vi "RunTest.vi"(8 "error in":errorcluster, 11 "Prueba31 in":refnum<class "Prueba31.lvclass">) -> (0 "error out":errorcluster, 2 "Resultado":string, 3 "Prueba31 out":refnum<class "Prueba31.lvclass">)   [LabVIEW 2019, in "Prueba31.lvclass"]
uses:
  Prueba31.lvclass
  Prueba31.lvclass/Prueba31.ctl
  QMH/Message Queue/Enqueue Message (Single).vi
  <vilib>/Utility/error.llb/Error Cluster From Error Code.vi
  RerenceAllControlsToolkit/_get control reference by name.vi
  <vilib>/ErrorRing/Error Ring.xnode
  QMH/Message Queue/Message Queue.lvlib
  QMH/User Event - Stop/User Event - Stop.lvlib
panel:
  in  "cb_frec_ext 2":string(combo)="31,5"
  in  "Tab Control":enum32{"externo", "interno"}(tab)
  out "cb_nivel_ext":dbl
  out "cb_frec_ext":dbl
  out "Tol - [dB]_ext":dbl
  out "Tol + [dB]_ext":dbl
  in  "generar_ext":bool
  out "cumple_ext":bool
  out "no_cumple_ext":bool
  out "frec_ref_ext":dbl
  out "nivel_ref_ext":dbl
  in  "señal_antes_ajuste_ext":dbl
  out "error_ext":dbl
  out "inc_expandida_ext":dbl
  in  "seguir_ext":bool
  out "voltaje_ext":dbl
  out "frecuencia_ext":dbl
  out "tipo gen_ext":string
  out "Tol - [dB]_int":dbl
  in  "cb_nivel_int":string(combo)="94"
  in  "cb_frec_int":string(combo)="31,5"
  out "Tol + [dB]_int":dbl
  out "cumple_int":bool
  out "no_cumple_int":bool
  out "frec_ref_int":dbl
  out "nivel_ref_int":dbl
  in  "señal_antes_ajuste_int":dbl
  out "error_int":dbl
  out "inc_expandida_int":dbl
  in  "seguir_int":bool
  out "tipo gen_int":string
  # "Elección Señal de Referencia \nsegún marca y modelo de sonómetro"
  # "Cumple"
  # "No Cumple"
  # "Tol - [dB]"
  # "Tol + [dB]"
  # "Frecuencia"
  # "Nivel"
  # "Frecuencia Señal de Referencia [Hz]"
  # "Nivel de Señal de Referencia [dB] (a)"
  # "Nivel de señal medida antes de ajuste [dB] (b)"
  # "Error [dB]"
  # "Incertidumbre Expandida ± [dB] (k=2)"
  # "1. Sensibilidad acústica absoluta. IEC 61252: 2002 Cláusula 6"
  # "Monitoreo"
  # "Frecuencia"
  # "Hz"
  # "Voltaje"
  # "V"
  # "Elección Señal de Referencia \nsegún marca y modelo de sonómetro"
  # "Cumple"
  # "No Cumple"
  # "Tol - [dB]"
  # "Tol + [dB]"
  # "Frecuencia"
  # "Nivel"
  # "Frecuencia Señal de Referencia [Hz]"
  # "Nivel de Señal de Referencia [dB] (a)"
  # "Nivel de señal medida antes de ajuste [dB] (b)"
  # "Error [dB]"
  # "Incertidumbre Expandida ± [dB] (k=2)"
  # "1. Sensibilidad acústica absoluta. IEC 61252: 2002 Cláusula 6"
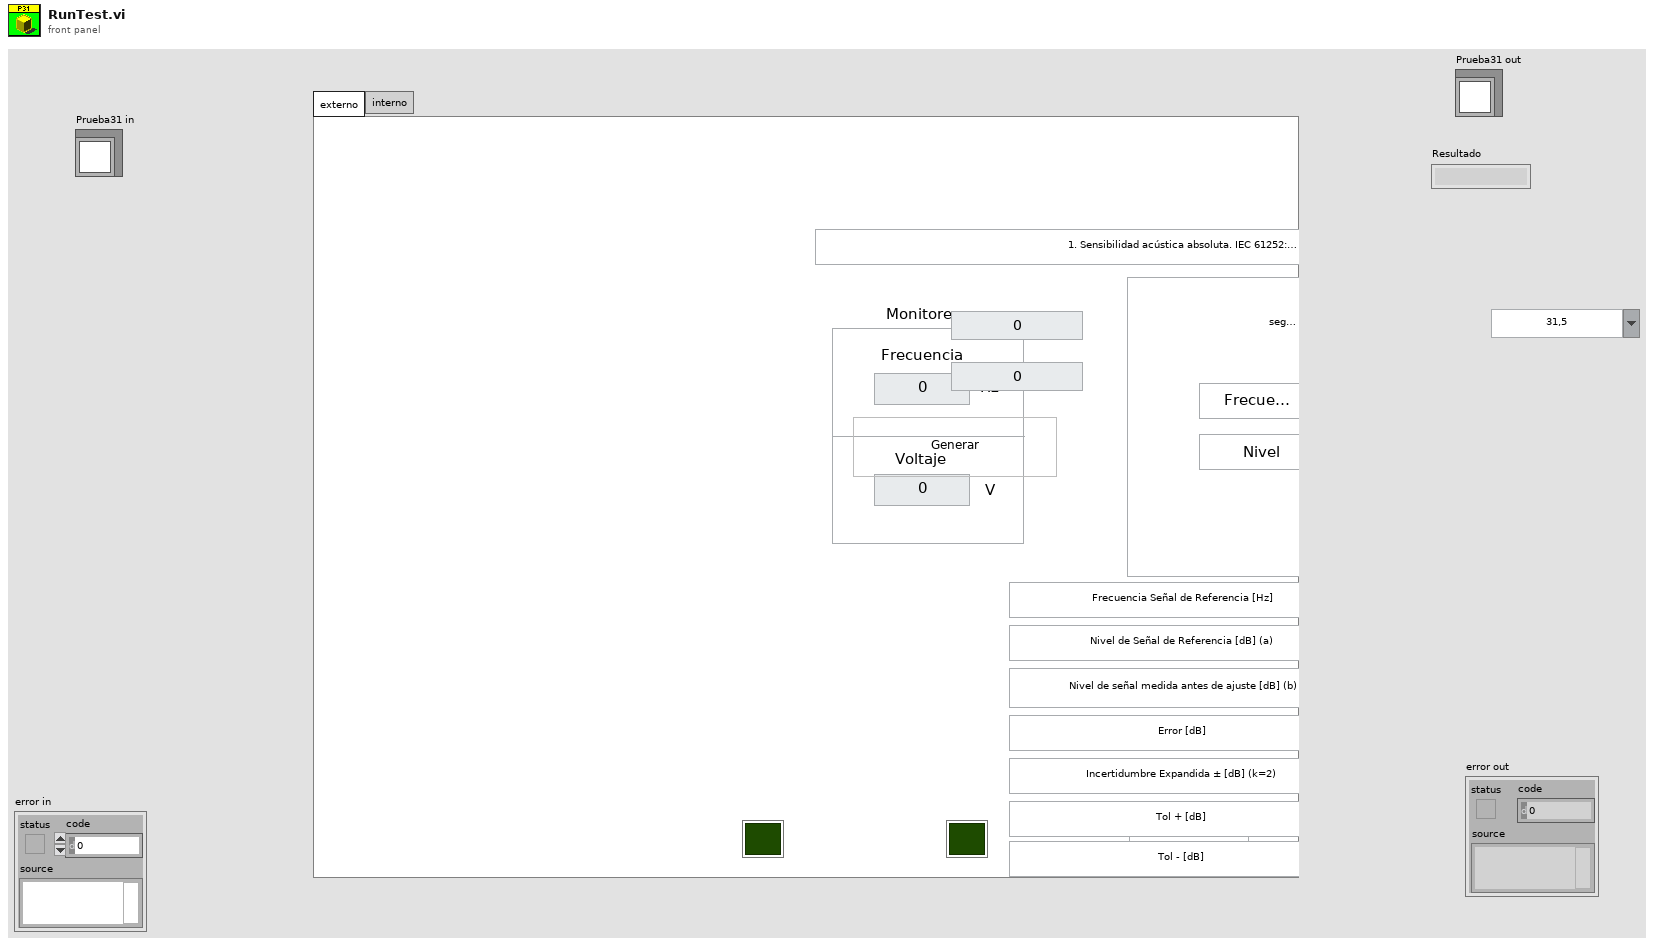
[diagram p1: front panel]
types:
  T1 = typedef "Message Queue.lvlib/All Message Queues.ctl" = cluster{"MHL":refnum<queue>, "Inst_CNT90":refnum<queue>, "Inst_DS360":refnum<queue>, "Inst_Keithley2002":refnum<queue>, "Inst_DAQ":refnum<queue>, "BD":refnum<queue>, "Pistofono":refnum<queue>, "Nexus":refnum<queue>}
  T2 = cluster{"ControlName":string, "ControlReference":refnum<vi>}[]
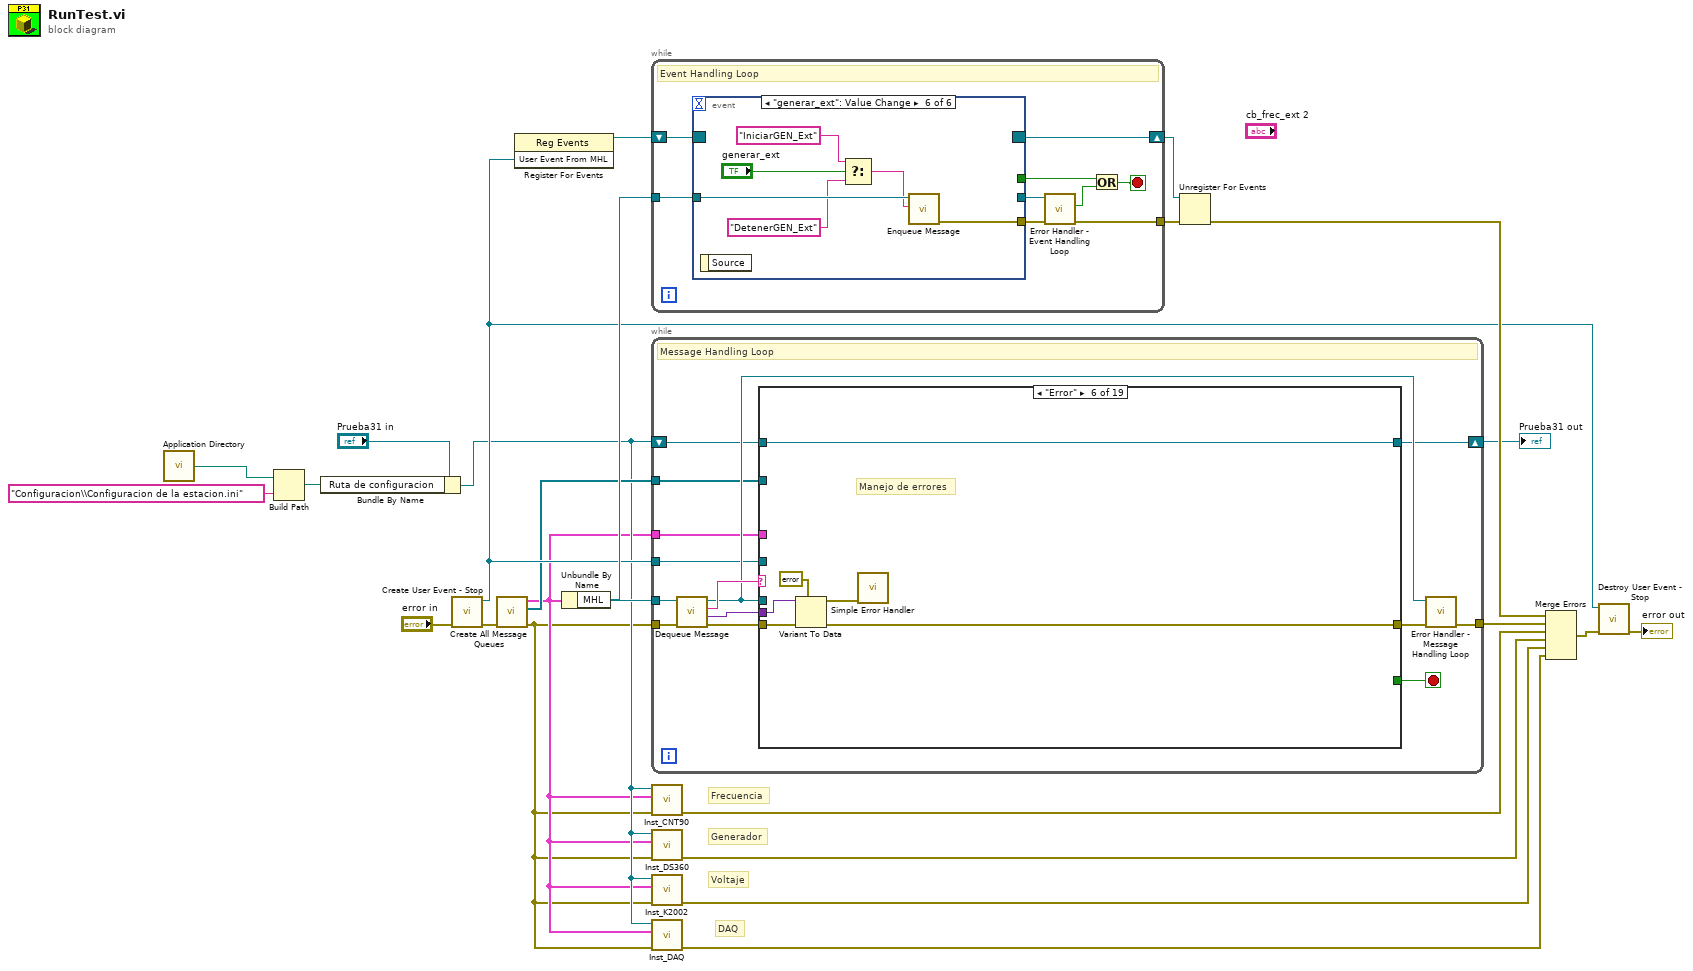
[diagram p0: block diagram]
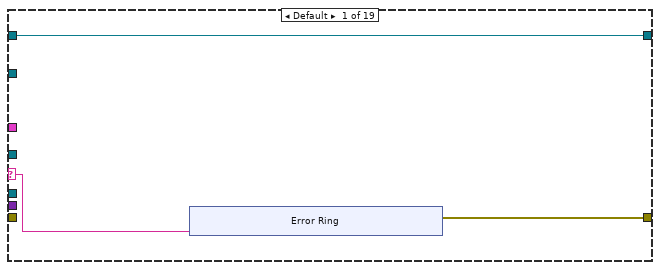
[diagram p2: hidden frame]
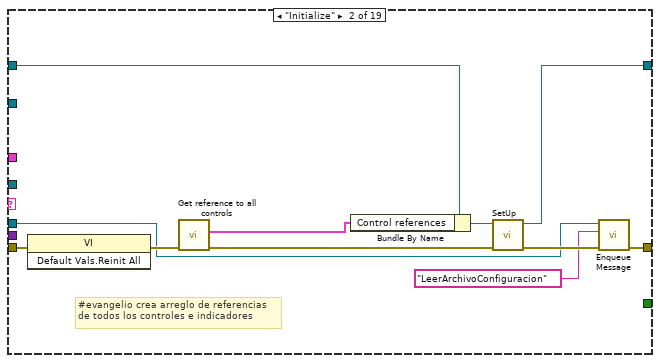
[diagram p3: hidden frame]
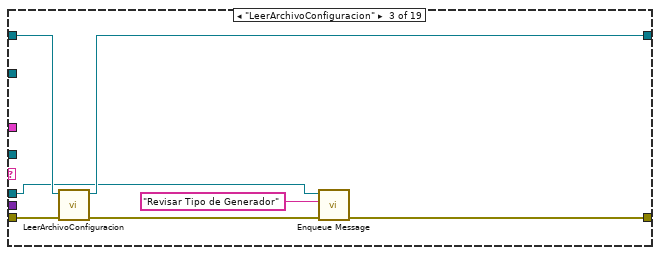
[diagram p4: hidden frame]
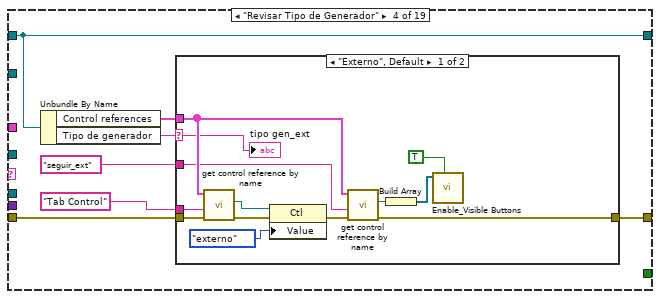
[diagram p5: hidden frame]
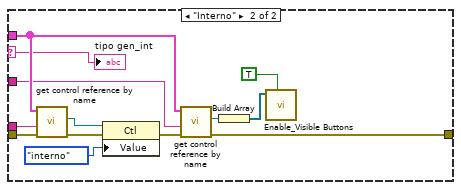
[diagram p6: hidden frame]
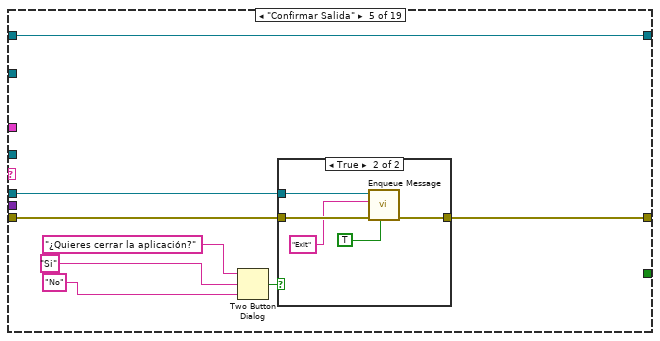
[diagram p7: hidden frame]
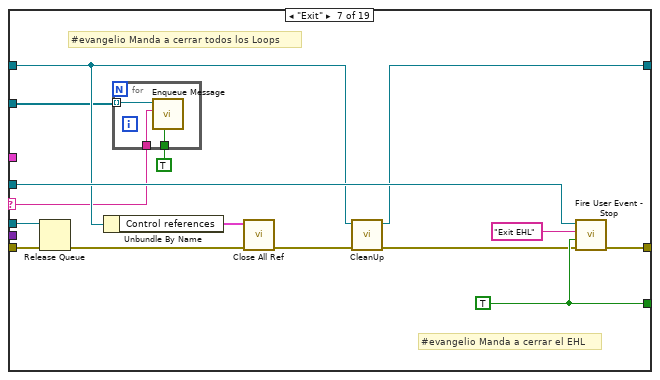
[diagram p9: hidden frame]
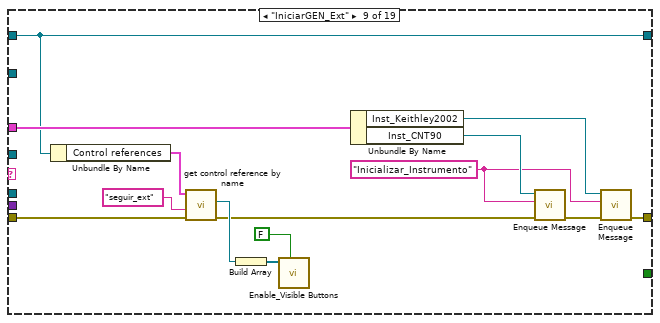
[diagram p11: hidden frame]
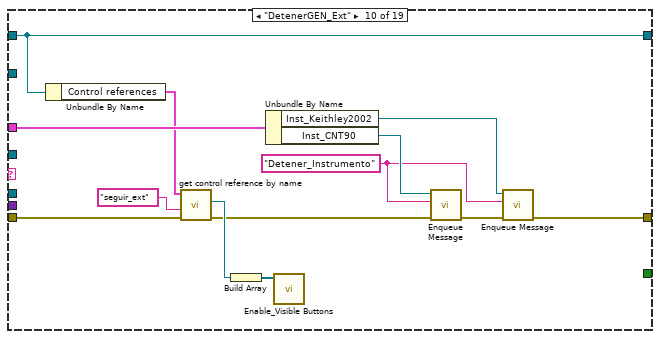
[diagram p12: hidden frame]
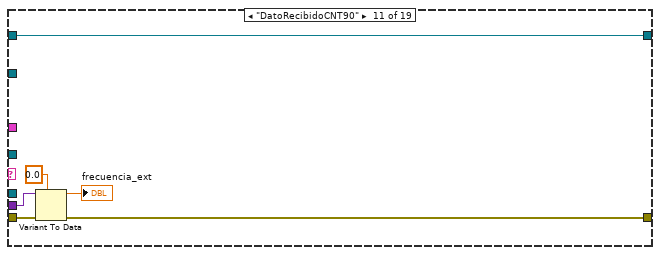
[diagram p13: hidden frame]
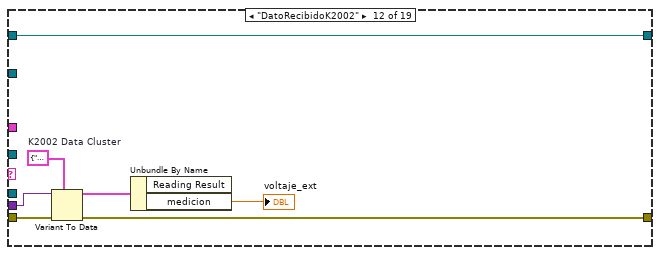
[diagram p14: hidden frame]
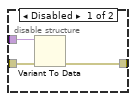
[diagram p16: hidden frame]
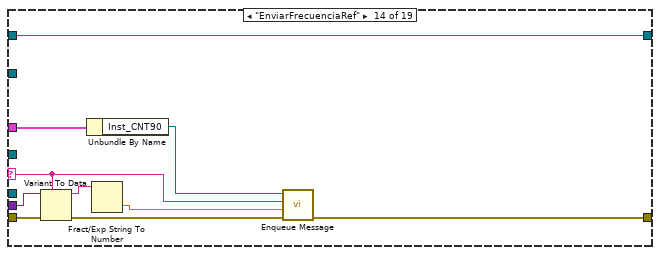
[diagram p17: hidden frame]
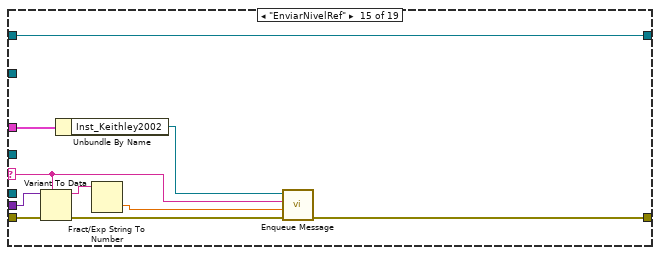
[diagram p18: hidden frame]
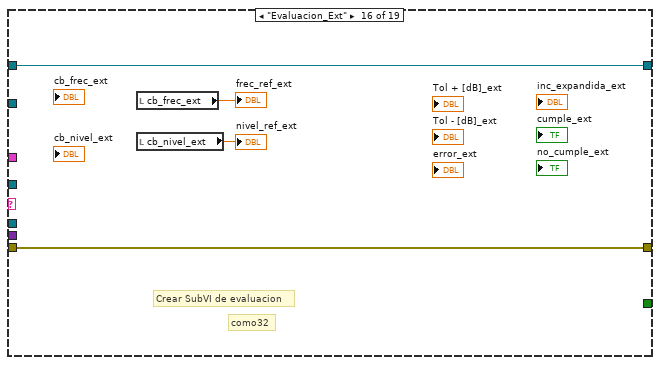
[diagram p19: hidden frame]
diagram:
  # "DAQ"
  # "Generador"
  # "Voltaje"
  # "Frecuencia"
  n1 = call <vilib>:"Application Directory.vi"() -> ("Application Directory"=w8:path)
  n2 = Build Path(base path=w8, name or relative path="Configuracion\\Configuracion de la estacion.ini") -> (appended path=w7:path)
  n3 = Bundle By Name(cluster="Prueba31 in", "Ruta de configuracion"=w7) -> (w4:refnum<class "Prueba31.lvclass">)
  n4 = call "Create User Event - Stop.vi"("error in (no error)"="error in") -> ("error out"=w21:errorcluster, "User Event From MHL"=w15:refnum<user-event>)  [unwired: 9 in]
  n5 = call "Create All Message Queues.vi"("error in (no error)"=w21) -> ("error out"=w2:errorcluster, "PL Queues Array"=w5:refnum<queue>[], "All Message Queues out"=w3:T1)  [unwired: 8 in]
  n6 = register-events(w15) -> (reference out=w24:refnum<event-registration>)  [unwired: 2 in, 1 out]
  n7 = Unbundle By Name(w3) -> ("MHL"=w20:refnum<queue>)
  n8 = while {
    tunnel: w20 -> [w33]
    tunnel: [w29] -> w23
    shift-right: [w31] -> w22
    shift-left: w24 -> [w32]
    stop <- w25 stop-if-true
    # "Event Handling Loop"
    n9 = event shown="[5] \"generar_ext\": Value Change" {
      selector: w32 -> [_ _ _ _ _ _]
      dyn-events: [_ _ _ _ _ _] -> w31
      timeout: _ -> [_ _ _ _ _ _]
      tunnel: w33 -> [w36 _ w47 w50 w53 w59]
      tunnel: [w38 _ w48 w51 w54 w60] -> w30
      tunnel: [w37 _ _ _ _ _] -> w28
      tunnel: [_ w39 _ _ _ _] -> w26
      event Panel Close? {
        w34 = TRUE
        n10 = event-data() -> ()  [unwired: 1 in, 1 out]
        n11 = call-poly "Enqueue Message.vi"("Priority Message? (F)"=w34, "Message"="Confirmar Salida", "Message Queue"=w36) -> ("error out"=w38:errorcluster, "dup Message Queue"=w37:refnum<queue>)  [unwired: 7 in]
        n12 = event-data("Discard?"=w34) -> ()  [unwired: 1 in, 1 out]
      }
      event User Event {
        n13 = event-data() -> ("User Event"=w41:string, "Event Data"=w40:variant)  [unwired: 1 in]
        n14 = case shown="\"Exit EHL\"" w41 {
          tunnel: w40 -> [_ w43]
          tunnel: [_ w42] -> w39
          frame Default {
          }
          frame "Exit EHL" {
            # "#evangelio Termina\nla ejecucion del EHL"
            n15 = Variant To Data(type=TRUE, Variant=w43) -> (data=w42:bool)  [unwired: 1 in, 1 out]
          }
        }
      }
      event "seguir_ext", "seguir_int": Value Change {
        n16 = event-data() -> ()  [unwired: 1 in, 1 out]
        n17 = call-poly "Enqueue Message.vi"("Priority Message? (F)"=TRUE, "Message"="Exit", "Message Queue"=w47) -> ("error out"=w48:errorcluster)  [unwired: 7 in, 1 out]
      }
      event "señal_antes_ajuste_ext": Value Change {
        n18 = event-data() -> ()  [unwired: 1 in, 1 out]
        n19 = call-poly "Enqueue Message.vi"("Message"="Evaluacion_Ext", "Message Queue"=w50) -> ("error out"=w51:errorcluster)  [unwired: 8 in, 1 out]
      }
      event "señal_antes_ajuste_int": Value Change {
        n20 = event-data() -> ()  [unwired: 1 in, 1 out]
        n21 = call-poly "Enqueue Message.vi"("Message"="Evaluacion_Int", "Message Queue"=w53) -> ("error out"=w54:errorcluster)  [unwired: 8 in, 1 out]
      }
      event "generar_ext": Value Change {
        n22 = event-data() -> ()  [unwired: 1 in, 1 out]
        n23 = Select(t="IniciarGEN_Ext" ("Message"), s="generar_ext", f="DetenerGEN_Ext" ("Message")) -> (s? t:f=w56:string)
        n24 = call-poly "Enqueue Message.vi"("Message"=w56, "Message Queue"=w59) -> ("error out"=w60:errorcluster)  [unwired: 8 in, 1 out]
      }
    }
    n25 = call "Error Handler - Event Handling Loop.vi"("error in (no error)"=w30, "Message Queue"=w28) -> ("dup error in"=w29:errorcluster, "Error?"=w27:bool)  [unwired: 7 in, 1 out]
    n26 = Or(x=w26, y=w27) -> (x .or. y?=w25:bool)
  }
  n27 = while {
    tunnel: w2 -> [w74]
    tunnel: w20 -> [w73]
    tunnel: [w67] -> w18
    shift-right: [w65] -> w16
    shift-left: w4 -> [w66]
    tunnel: w3 -> [w63]
    tunnel: w15 -> [w62]
    tunnel: w5 -> [w61]
    stop <- w64 stop-if-true
    # "Message Handling Loop"
    n28 = call "Dequeue Message.vi"("error in (no error)"=w74, "Message Queue"=w73) -> ("error out"=w70:errorcluster, "Message Data"=w71:variant, "Message"=w72:string, "dup Message Queue"=w69:refnum<queue>)  [unwired: 6 in]
    n29 = case shown="\"Error\"" w72 {
      selector: w72 -> [w76 _ _ _ _ _ w158 _ _ _ _ _ _ w224 w234 _ _ _ _]
      tunnel: w69 -> [_ w88 w97 _ w136 _ w169 _ _ _ _ _ _ _ _ _ _ _ _]
      tunnel: w71 -> [_ _ _ _ _ w151 _ _ _ _ w205 w212 w216 w231 w241 _ _ _ _]
      tunnel: w70 -> [_ w95 w102 w106 w142 w152 w168 w175 w177 w199 w206 w213 w217 w232 w242 w247 w249 w255 w257]
      tunnel: [w75 w89 w98 w103 w141 w153 w166 w175 w184 w192 w207 w214 w218 w228 w238 w247 w249 w255 w257] -> w68
      tunnel: w66 -> [w77 w93 w101 w105 w143 w155 w159 w174 w179 w200 w208 w215 w219 w233 w243 w246 w248 w254 w256]
      tunnel: [w77 w91 w100 w105 w143 w155 w160 w174 w179 w200 w208 w215 w219 w233 w243 w246 w248 w254 w256] -> w65
      tunnel: [_ _ _ _ _ _ w163 _ _ _ _ _ _ _ _ _ _ _ _] -> w64
      tunnel: w63 -> [_ _ _ _ _ _ _ _ w189 w202 _ _ _ w226 w236 _ _ _ _]
      tunnel: w62 -> [_ _ _ _ _ _ w165 _ _ _ _ _ _ _ _ _ _ _ _]
      tunnel: w61 -> [_ _ _ _ _ _ w156 _ _ _ _ _ _ _ _ _ _ _ _]
      frame Default {
        n30 = xnode "Error Ring"("parameter 0"=w76) -> ("error out"=w75:errorcluster)
      }
      frame "Initialize" {
        # "#evangelio crea arreglo de referencias\nde todos los controles e indicadores"
        n31 = invoke class="VI" method="Default Vals.Reinit All"(error in=w95) -> (error out=w94:errorcluster)  [unwired: 2 in, 2 out]
        n32 = call "Get reference to all controls.vi"("error in (no error)"=w94) -> ("error out"=w85:errorcluster, "Control references"=w86:T2)  [unwired: 5 in]
        n33 = Bundle By Name(cluster=w93, "Control references"=w86) -> (w92:refnum<class "Prueba31.lvclass">)
        n34 = call-dynamic "SetUp.vi"("error in (no error)"=w85, "Prueba08 in"=w92) -> ("error out"=w90:errorcluster, "Prueba08 out"=w91:refnum<class "Prueba31.lvclass">)  [unwired: 8 in]
        n35 = call-poly "Enqueue Message.vi"("error in (no error)"=w90, "Message"="LeerArchivoConfiguracion", "Message Queue"=w88) -> ("error out"=w89:errorcluster)  [unwired: 7 in, 1 out]
      }
      frame "LeerArchivoConfiguracion" {
        n36 = call "LeerArchivoConfiguracion.vi"("error in"=w102, "Prueba31 in"=w101) -> ("error out"=w99:errorcluster, "Prueba31 out"=w100:refnum<class "Prueba31.lvclass">)  [unwired: 8 in]
        n37 = call-poly "Enqueue Message.vi"("error in (no error)"=w99, "Message"="Revisar Tipo de Generador", "Message Queue"=w97) -> ("error out"=w98:errorcluster)  [unwired: 7 in, 1 out]
      }
      frame "Revisar Tipo de Generador" {
        n38 = Unbundle By Name(w105) -> ("Control references"=w108:T2, "Tipo de generador"=w109:string)
        n39 = case shown="\"Externo\", Default" w109 {
          selector: w109 -> [w110 w123]
          tunnel: w106 -> [w122 w135]
          tunnel: w108 -> [w117 w130]
          tunnel: "Tab Control" -> [w121 w134]
          tunnel: "seguir_ext" -> [w111 w124]
          tunnel: [w113 w126] -> w103
          frame "Externo", Default {
            n40 = call-poly "get control reference by name.vi"("error in (no error)"=w122, "Control name"=w121, "Control references"=w117) -> ("error out"=w119:errorcluster, "Ctl Refnum"=w120:refnum<vi>)  [unwired: 3 in]
            n41 = property class="Ctl"(reference=w120, error in=w119, "Value"=enum32{"externo", "interno"}."externo" ("Tab Control")) -> (error out=w116:errorcluster)  [unwired: 1 out]
            n42 = call-poly "get control reference by name.vi"("error in (no error)"=w116, "Control name"=w111, "Control references"=w117) -> ("error out"=w113:errorcluster, "Ctl Refnum"=w115:refnum<vi>)  [unwired: 3 in]
            n43 = Build Array(w115) -> (w114:refnum<vi>[])
            n44 = call "Enable_Visible Buttons.vi"("Enable? (T)"=TRUE, "Controls Ref Array"=w114) -> ()  [unwired: 10 in]
            "tipo gen_ext" <- w110
          }
          frame "Interno" {
            n45 = call-poly "get control reference by name.vi"("error in (no error)"=w135, "Control name"=w134, "Control references"=w130) -> ("error out"=w132:errorcluster, "Ctl Refnum"=w133:refnum<vi>)  [unwired: 3 in]
            n46 = property class="Ctl"(reference=w133, error in=w132, "Value"=enum32{"externo", "interno"}."interno" ("Tab Control")) -> (error out=w129:errorcluster)  [unwired: 1 out]
            n47 = call-poly "get control reference by name.vi"("error in (no error)"=w129, "Control name"=w124, "Control references"=w130) -> ("error out"=w126:errorcluster, "Ctl Refnum"=w128:refnum<vi>)  [unwired: 3 in]
            n48 = Build Array(w128) -> (w127:refnum<vi>[])
            n49 = call "Enable_Visible Buttons.vi"("Enable? (T)"=TRUE, "Controls Ref Array"=w127) -> ()  [unwired: 10 in]
            "tipo gen_int" <- w123
          }
        }
      }
      frame "Confirmar Salida" {
        n50 = Two Button Dialog(message="¿Quieres cerrar la aplicación?", 1:"No" ("T button name (\"OK\")"), 2:"Si" ("T button name (\"OK\")")) -> (T button?=w137:bool)
        n51 = case shown="True" w137 {
          tunnel: w142 -> [w144 w149]
          tunnel: [w144 w148] -> w141
          tunnel: w136 -> [_ w147]
          frame False {
          }
          frame True {
            n52 = call-poly "Enqueue Message.vi"("Priority Message? (F)"=TRUE, "error in (no error)"=w149, "Message"="Exit", "Message Queue"=w147) -> ("error out"=w148:errorcluster)  [unwired: 6 in, 1 out]
          }
        }
      }
      frame "Error" {
        # "Manejo de errores"
        n53 = Variant To Data(error in=w152, type=errorcluster {"status"=FALSE, "code"=0, "source"=""} ("error constant"), Variant=w151) -> (data=w150:errorcluster, error out=w153:errorcluster)
        n54 = call <vilib>:"Simple Error Handler.vi"("error in (no error)"=w150) -> ()  [unwired: 4 in, 5 out]
      }
      frame "Exit" {
        w163 = TRUE
        # "#evangelio Manda a cerrar el EHL"
        # "#evangelio Manda a cerrar todos los Loops"
        n55 = Release Queue(queue=w169, error in (no error)=w168) -> (error out=w167:errorcluster)  [unwired: 1 in, 2 out]
        n56 = Unbundle By Name(w159) -> ("Control references"=w170:T2)
        n57 = for {
          tunnel: w156 -> [w173] mode=indexing
          tunnel: w158 -> [w172]
          tunnel: TRUE -> [w171]
          n58 = call-poly "Enqueue Message.vi"("Priority Message? (F)"=w171, "Message"=w172, "Message Queue"=w173) -> ()  [unwired: 7 in, 2 out]
        }
        n59 = call "Close All Ref.vi"("error in (no error)"=w167, "Control references"=w170) -> ("error out"=w162:errorcluster)  [unwired: 9 in]
        n60 = call-dynamic "CleanUp.vi"("error in (no error)"=w162, "Prueba08 in"=w159) -> ("error out"=w161:errorcluster, "Prueba08 out"=w160:refnum<class "Prueba31.lvclass">)  [unwired: 8 in]
        n61 = call "Fire User Event - Stop.vi"("error in (no error)"=w161, "Event Data"=w163, "User Event"="Exit EHL", "User Event in"=w165) -> ("error out"=w166:errorcluster)  [unwired: 7 in]
      }
      frame "---- EXT ----" {
      }
      frame "IniciarGEN_Ext" {
        w185 = "Inicializar_Instrumento" ("Message")
        n62 = Unbundle By Name(w179) -> ("Control references"=w180:T2)
        n63 = call-poly "get control reference by name.vi"("error in (no error)"=w177, "Control name"="seguir_ext", "Control references"=w180) -> ("error out"=w178:errorcluster, "Ctl Refnum"=w182:refnum<vi>)  [unwired: 3 in]
        n64 = Build Array(w182) -> (w181:refnum<vi>[])
        n65 = call "Enable_Visible Buttons.vi"("Enable? (T)"=FALSE, "Controls Ref Array"=w181) -> ()  [unwired: 10 in]
        n66 = Unbundle By Name(w189) -> ("Inst_Keithley2002"=w186:refnum<queue>, "Inst_CNT90"=w188:refnum<queue>)
        n67 = call-poly "Enqueue Message.vi"("error in (no error)"=w178, "Message"=w185, "Message Queue"=w188) -> ("error out"=w187:errorcluster)  [unwired: 7 in, 1 out]
        n68 = call-poly "Enqueue Message.vi"("error in (no error)"=w187, "Message"=w185, "Message Queue"=w186) -> ("error out"=w184:errorcluster)  [unwired: 7 in, 1 out]
      }
      frame "DetenerGEN_Ext" {
        w190 = "Detener_Instrumento" ("Message")
        n69 = Unbundle By Name(w200) -> ("Control references"=w195:T2)
        n70 = call-poly "get control reference by name.vi"("error in (no error)"=w199, "Control name"="seguir_ext", "Control references"=w195) -> ("error out"=w194:errorcluster, "Ctl Refnum"=w197:refnum<vi>)  [unwired: 3 in]
        n71 = Build Array(w197) -> (w196:refnum<vi>[])
        n72 = Unbundle By Name(w202) -> ("Inst_Keithley2002"=w191:refnum<queue>, "Inst_CNT90"=w201:refnum<queue>)
        n73 = call "Enable_Visible Buttons.vi"("Controls Ref Array"=w196) -> ()  [unwired: 11 in]
        n74 = call-poly "Enqueue Message.vi"("error in (no error)"=w194, "Message"=w190, "Message Queue"=w201) -> ("error out"=w193:errorcluster)  [unwired: 7 in, 1 out]
        n75 = call-poly "Enqueue Message.vi"("error in (no error)"=w193, "Message"=w190, "Message Queue"=w191) -> ("error out"=w192:errorcluster)  [unwired: 7 in, 1 out]
      }
      frame "DatoRecibidoCNT90" {
        n76 = Variant To Data(error in=w206, type=0.0, Variant=w205) -> (data=→"frecuencia_ext":dbl, error out=w207:errorcluster)
      }
      frame "DatoRecibidoK2002" {
        w211 = cluster{"Reading Result":string, "medicion":dbl} {"Reading Result"="", "medicion"=0.0}  # K2002 Data Cluster
        n77 = Variant To Data(error in=w213, type=w211, Variant=w212) -> (data=w210:cluster{"Reading Result":string, "medicion":dbl}, error out=w214:errorcluster)
        n78 = Unbundle By Name(w210) -> ("medicion"=→"voltaje_ext":dbl)  [unwired: 1 out]
      }
      frame "DatoRecibidoDS360" {
        n79 = disable-structure shown="Enabled" {
          disable-tunnel: [w222 w223] -> w218
          disable-tunnel: w217 -> [w221 w223]
          disable-tunnel: w216 -> [w220 _]
          frame Disabled {
            n80 = Variant To Data(error in=w221, Variant=w220) -> (error out=w222:errorcluster)  [unwired: 1 in, 1 out]
          }
          frame Enabled {
          }
        }
      }
      frame "EnviarFrecuenciaRef" {
        n81 = Variant To Data(error in=w232, type=w224, Variant=w231) -> (data=w230:string, error out=w229:errorcluster)
        n82 = Unbundle By Name(w226) -> ("Inst_CNT90"=w225:refnum<queue>)
        n83 = Fract/Exp String To Number(string=w230) -> (number=w227:dbl)  [unwired: 3 in, 1 out]
        n84 = call-poly "Enqueue Message.vi"("error in (no error)"=w229, "Message Data"=w227, "Message"=w224, "Message Queue"=w225) -> ("error out"=w228:errorcluster)  [unwired: 6 in, 1 out]
      }
      frame "EnviarNivelRef" {
        n85 = Variant To Data(error in=w242, type=w234, Variant=w241) -> (data=w240:string, error out=w239:errorcluster)
        n86 = Unbundle By Name(w236) -> ("Inst_Keithley2002"=w235:refnum<queue>)
        n87 = Fract/Exp String To Number(string=w240) -> (number=w237:dbl)  [unwired: 3 in, 1 out]
        n88 = call-poly "Enqueue Message.vi"("error in (no error)"=w239, "Message Data"=w237, "Message"=w234, "Message Queue"=w235) -> ("error out"=w238:errorcluster)  [unwired: 6 in, 1 out]
      }
      frame "Evaluacion_Ext" {
        # "como32"
        # "Crear SubVI de evaluacion"
        n89 = local read "cb_frec_ext"() -> (→"frec_ref_ext":dbl)
        n90 = local read "cb_nivel_ext"() -> (→"nivel_ref_ext":dbl)
      }
      frame "---- INT ----" {
      }
      frame "Evaluacion_Int" {
        # "Crear SubVI de evaluacion"
        n91 = Fract/Exp String To Number(string="cb_frec_int") -> (number=→"frec_ref_int":dbl)  [unwired: 3 in, 1 out]
        n92 = Fract/Exp String To Number(string="cb_nivel_int") -> (number=→"nivel_ref_int":dbl)  [unwired: 3 in, 1 out]
      }
      frame "--------------------------Contoles---------------------------" {
      }
    }
    n93 = call "Error Handler - Message Handling Loop.vi"("error in (no error)"=w68, "Message Queue"=w69) -> ("dup error in"=w67:errorcluster)  [unwired: 8 in, 1 out]
  }
  "Prueba31 out" <- w16
  n94 = call "Inst_CNT90.vi"("error in"=w2, "All Message Queues in"=w3, "Prueba31 in"=w4) -> ("error out"=w12:errorcluster)  [unwired: 8 in]
  n95 = call "Inst_DS360.vi"("error in"=w2, "All Message Queues in"=w3, "Prueba31 in"=w4) -> ("error out"=w11:errorcluster)  [unwired: 8 in]
  n96 = call "Inst_K2002.vi"("error in"=w2, "All Message Queues in"=w3, "Prueba31 in"=w4) -> ("error out"=w10:errorcluster)  [unwired: 8 in]
  n97 = call "Inst_DAQ.vi"("error in"=w2, "All Message Queues in"=w3, "Prueba31 in"=w4) -> ("error out"=w1:errorcluster)  [unwired: 8 in]
  n98 = Unregister For Events(event registration refnum=w22, error in=w23) -> (error out=w19:errorcluster)
  n99 = Merge Errors(w19, w18, w12, w11, w10, w1) -> (w17:errorcluster)
  n100 = call "Destroy User Event - Stop.vi"("error in (no error)"=w17, "User Event"=w15) -> ("error out"=→"error out":errorcluster)  [unwired: 9 in]
